vi "RingControls - NoTypeDefs.vi"(4 "Text Ring (U64)":u64(ring)=13746784023709451617 items=["Value 1"=18146734073709511613, "Value 2"=14946714073719251615, "Value 3"=13746784023709451617, "Value 4"=15946764073709551611, "Value 5"=17146744071709251618], 5 "Enum":enum32{"AAA", "BBB", "CCCC", "DDDD", "EEEE"}(ring)=enum."DDDD", 6 "Numeric Constants":dbl(ring)=3.141593 format="%#.6f" items=["NegativeInfinity"=-inf, "Pi"=3.141593, "NaturalLogarithmBase"=2.718282, "MolarGasConstant"=8.314472, "SpeedOfLightInVacuum "=299792458.0, "RydbergConstant"=10973731.568527, "NotANumber"=nan, "PostitiveInfinity"=inf], 7 "Menu Ring":i16(ring)=330 items=["Menu Item 1"=12, "Menu Item 2"=-45, "Menu Item 3"=150, "Menu Item 4"=330, "Menu Item 5"=-455], 8 "Text Ring (Float64)":sgl(ring)=5566.0 items=["Text Ring Value 1"=-1.231231e+08, "Text Ring Value 2"=2233, "Text Ring Value 3"=4455, "Text Ring Value 4"=5566, "Text Ring Value 5"=7788], 9 "Text & Pict Ring":i32(ring)=2233 items=["Text & Pict Ring 1"=1122, "Text & Pict Ring 2"=2233, "Text & Pict Ring 3"=3344, "Text & Pict Ring 4"=4455, "Text & Pict Ring 5"=5566], 10 "Pict Ring Control":u16(ring)=2, 11 "Text Ring":i8(ring)=-66 items=["Text Ring Value 1"=111, "Text Ring Value 2"=-71, "Text Ring Value 3"=103, "Text Ring Value 4"=-66, "Text Ring Value 5"=108]) -> ()   [LabVIEW 2012]
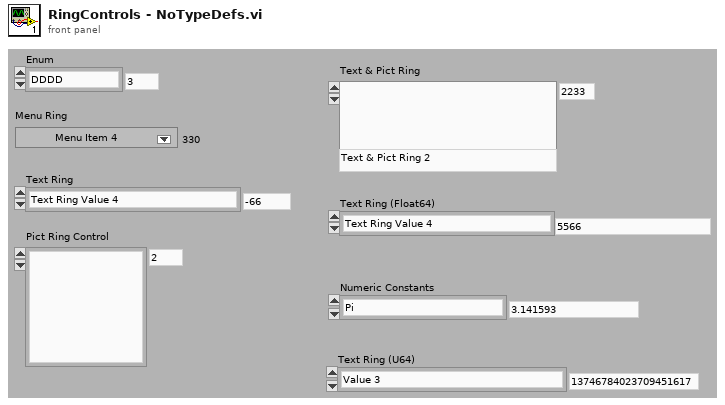
[diagram p1: front panel]
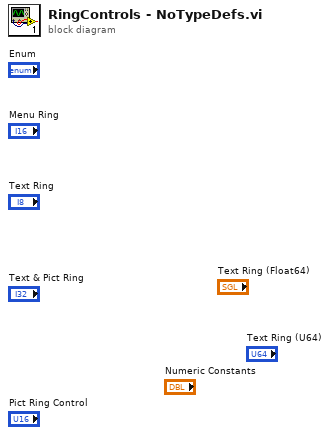
[diagram p0: block diagram]
diagram:
